vi "CRDS Main.vi"() -> ()   [LabVIEW 2015, in "CRDS.lvclass"]
doc: "This is a basic template for using with children of the instrument class. This provides the basic functionality in a queued state machine. Since the instrument class is abstract, the class must be filled out for meaningful functionality. To get desired behavior, simply swap the instrument class constant in the VIT with a child class that has been properly populated."
uses:
  Main/CRDS.lvclass
  Data/Cell/extparam.ctl
  <vilib>/Utility/error.llb/DialogType.ctl
  Instrument/state.ctl
  Data/Cell/CRDS Cell Data.lvclass/CRDS Cell Data.ctl
  Data/Cell/Read extParam.vi
  <vilib>/Analysis/1siggen.llb/Ramp Pattern by Delta.vi
  Main/Read Data.vi
  Data/Main/Read CellData.vi
  Data/Main/CRDS Data.lvclass
  Data/Cell/CRDS Cell Data.lvclass
  Instrument/Instrument.lvclass
  <vilib>/Analysis/NI_AALBase.lvlib
panel:
  in  "ExpData In":cluster{"A":dbl, "B":dbl, "tau":dbl}[](array[cluster])=[{"A"=16000.0, "B"=100.0, "tau"=60.0}, {"A"=16000.0, "B"=100.0, "tau"=20.0}, {"A"=16000.0, "B"=100.0, "tau"=180.0}]
  out "ExtData":T1[](array[typedef])
  out "taus":cluster{"[0]":dbl, "[1]":dbl, "[2]":dbl}(graph)
  out "tau calc":u32
  in  "Filter":bool
  in  "HK Data":dbl[](array[numeric])
  out "tau_gen":u32
  in  "stop":bool
  out "HK Data":cluster{"[0]":dbl, "[1]":dbl}(graph)
  out "RD Data":dbl[][](graph)
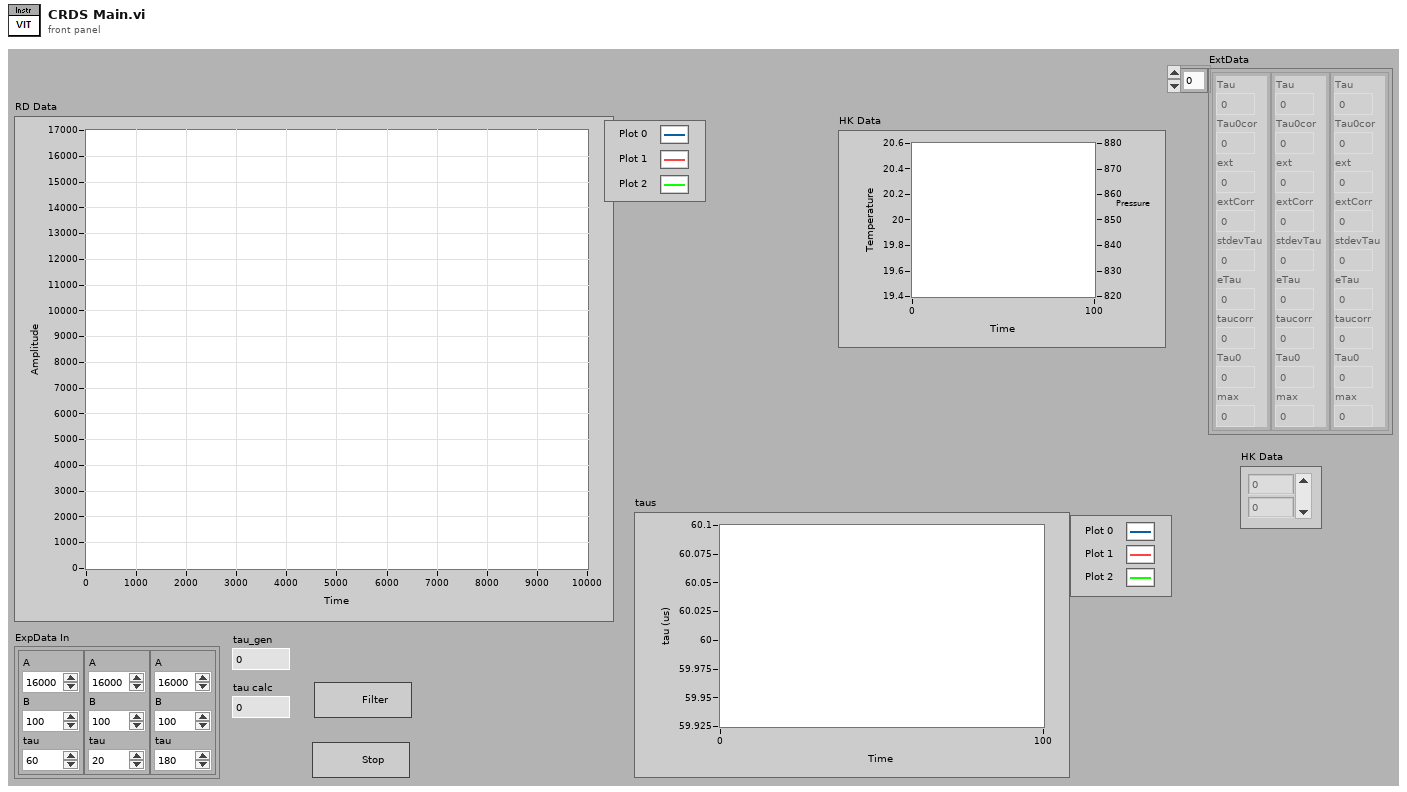
[diagram p1: front panel]
types:
  T1 = typedef "extparam.ctl" = cluster{"Tau":sgl, "Tau0cor":sgl, "ext":sgl, "extCorr":sgl, "stdevTau":sgl, "eTau":sgl, "taucorr":sgl, "Tau0":sgl, "max":sgl}
  T2 = typedef "Instrument.lvclass/state.ctl" = enum8{"Configure", "Acquire", "Wait", "Quit", "Handle Error", "NOOP"}
  T3 = typedef "DialogType.ctl" = u16
  T4 = cluster{"RD Data":dbl[][], "HK Data":dbl[], "Filter":bool}
  T5 = cluster{"RD Data Out":dbl[][], dbl[], "Filter":bool}
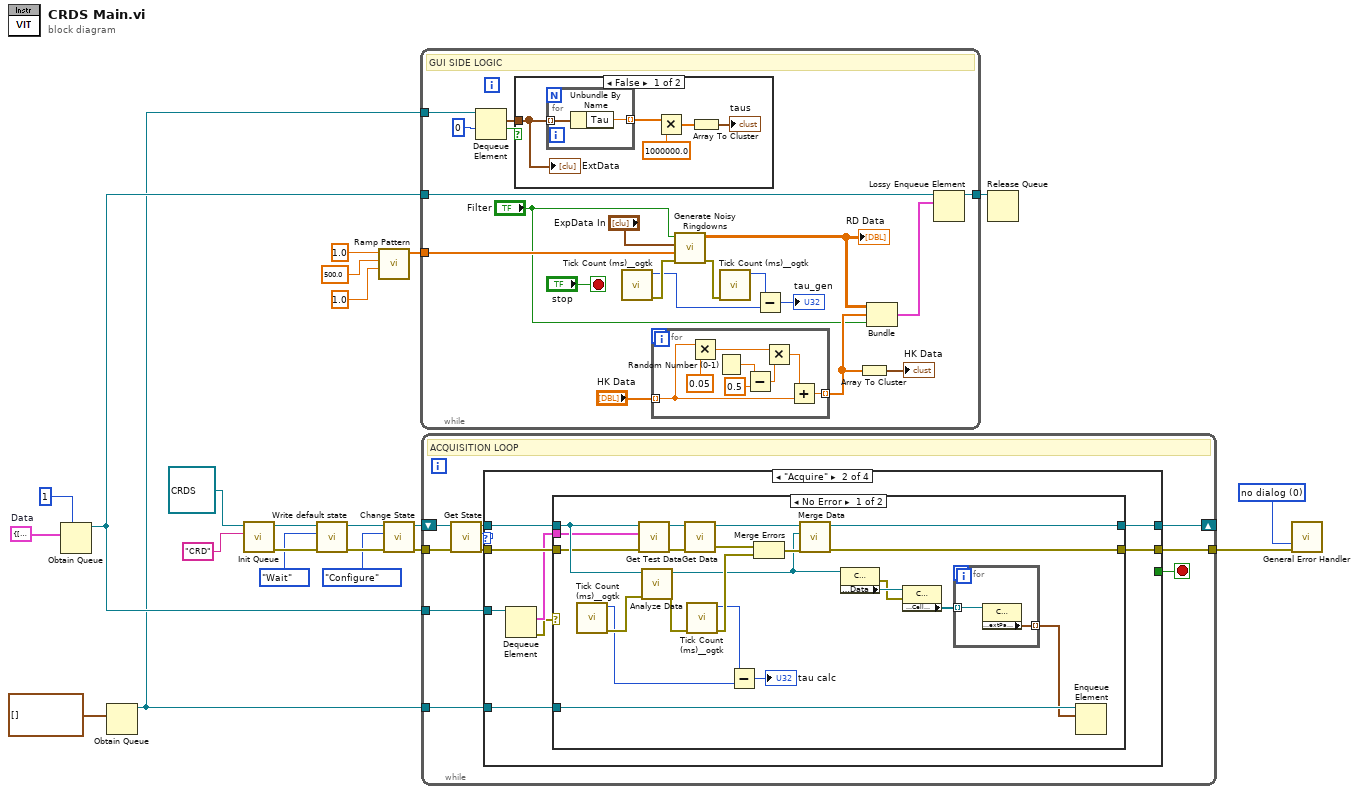
[diagram p0: block diagram]
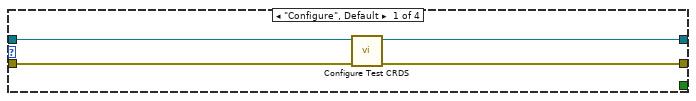
[diagram p2: hidden frame]
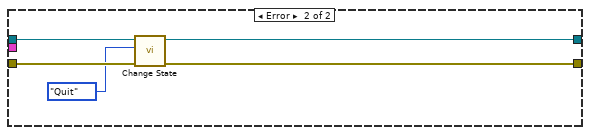
[diagram p3: hidden frame]
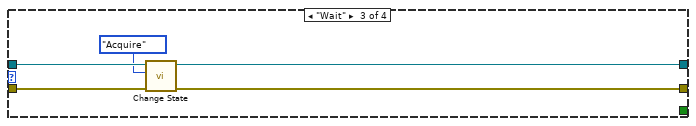
[diagram p4: hidden frame]
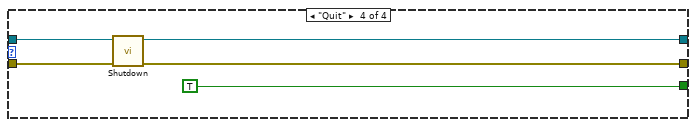
[diagram p5: hidden frame]
diagram:
  w16 = T3 0 items=["no dialog", "OK message", "continue or stop message", "OK message + warnings", "continue/stop + warnings"] ("type of dialog (OK msg:1)")
  w18 = T4 {"RD Data"=[], "HK Data"=[], "Filter"=FALSE}  # Data
  n1 = Obtain Queue(max queue size (-1, unlimited)=1, element data type=w18) -> (queue out=w13:refnum<queue>)  [unwired: 3 in, 2 out]
  n2 = Obtain Queue(element data type=T1[] []) -> (queue out=w1:refnum<queue>)  [unwired: 4 in, 2 out]
  n3 = call "Init Queue.vi"("queue_name"="CRD", "Instrument in"=refnum<class "CRDS.lvclass"> refnum ("CRDS")) -> ("error out"=w10:errorcluster, "Instrument out"=w11:refnum<class "CRDS.lvclass">)  [unwired: 8 in]
  n4 = call "Write default state.vi"("error in (no error)"=w10, "instr state"=state."Wait", "Instrument in"=w11) -> ("error out"=w6:errorcluster, "Instrument out"=w8:refnum<class "CRDS.lvclass">)  [unwired: 7 in]
  n5 = call-poly <vilib>:"Ramp Pattern.vi"("start"=1.0, "end"=500.0, "delta"=1.0) -> ("Ramp Pattern"=w19:dbl[])  [unwired: 6 in, 2 out]
  n6 = call "Change State.vi"("error in"=w6, "instr state"=state."Configure", "Instrument in"=w8) -> ("error out"=w5:errorcluster, "Instrument out"=w7:refnum<class "CRDS.lvclass">)  [unwired: 7 in]
  n7 = while {
    tunnel: w19 -> [w42]
    tunnel: w13 -> [w36]
    tunnel: [w31] -> w12
    tunnel: w1 -> [w28]
    stop <- "stop" stop-if-true
    # "GUI SIDE LOGIC"
    n8 = Dequeue Element(queue=w28, timeout in ms (-1)=0) -> (element=w25:T1[], timed out?=w26:bool)  [unwired: 1 in, 2 out]
    n9 = case shown="False" w26 {
      tunnel: w25 -> [w47 _]
      frame False {
        n10 = for {
          tunnel: w47 -> [w49] mode=indexing
          tunnel: [w48] -> w45 mode=indexing
          n11 = Unbundle By Name(w49) -> ("Tau"=w48:sgl)
        }
        n12 = Multiply(x=w45, y=1000000.0) -> (x*y=w43:dbl[])
        n13 = Array To Cluster(array=w43) -> (cluster=→"taus":cluster{"[0]":dbl, "[1]":dbl, "[2]":dbl})
        "ExtData" <- w47
      }
      frame True {
      }
    }
    n14 = call <userlib>:"Tick Count (ms)__ogtk.vi"() -> ("error out"=w41:errorcluster, "millisecond timer value"=w38:u32)  [unwired: 10 in]
    n15 = for {
      tunnel: "HK Data" -> [w51] mode=indexing
      tunnel: [w50] -> w30 mode=indexing
      n16 = Multiply(x=w51, y=0.05) -> (x*y=w53:dbl)
      n17 = Random Number (0-1)() -> (number: 0 to 1=w56:dbl)
      n18 = Subtract(x=w56, y=0.5) -> (x-y=w54:dbl)
      n19 = Multiply(x=w53, y=w54) -> (x*y=w52:dbl)
      n20 = Add(x=w52, y=w51) -> (x+y=w50:dbl)
    }
    n21 = call "Generate Noisy Ringdowns.vi"("error in"=w41, "Ramp Pattern"=w42, "ExpData In"="ExpData In", "Filter"="Filter") -> ("error out"=w40:errorcluster, "RD Data Out"=w35:dbl[][])  [unwired: 6 in]
    "RD Data" <- w35
    n22 = call <userlib>:"Tick Count (ms)__ogtk.vi"("error in (no error)"=w40) -> ("millisecond timer value"=w39:u32)  [unwired: 9 in, 1 out]
    n23 = Subtract(x=w39, y=w38) -> (x-y=→"tau_gen":u32)
    n24 = Array To Cluster(array=w30) -> (cluster=→"HK Data":cluster{"[0]":dbl, "[1]":dbl})
    n25 = Bundle("RD Data Out"=w35, w30, "Filter"="Filter") -> (w33:T5)  [unwired: 1 in]
    n26 = Lossy Enqueue Element(queue=w36, element=w33) -> (queue out=w31:refnum<queue>)  [unwired: 1 in, 3 out]
  }
  n27 = while "Acquisition" {
    tunnel: w5 -> [w67]
    shift-right: [w61] -> _
    shift-left: w7 -> [w65]
    tunnel: [w60] -> w17
    tunnel: w13 -> [w59]
    tunnel: w1 -> [w58]
    stop <- w62 stop-if-true
    # "ACQUISITION LOOP"
    n28 = call "Get State.vi"("error in"=w67, "Instrument in"=w65) -> ("error out"=w63:errorcluster, "default state"=w66:T2, "Instrument out"=w64:refnum<class "CRDS.lvclass">)  [unwired: 7 in]
    n29 = case shown="\"Acquire\"" w66 {
      tunnel: w64 -> [w71 w76 w113 w117]
      tunnel: w63 -> [w70 w79 w112 w116]
      tunnel: [_ _ _ TRUE] -> w62
      tunnel: [w69 w78 w111 w115] -> w61
      tunnel: [w68 w77 w110 w114] -> w60
      tunnel: w59 -> [_ w75 _ _]
      tunnel: w58 -> [_ w72 _ _]
      frame "Configure", Default {
        n30 = call "Configure Test CRDS.vi"("error in (no error)"=w70, "CRDS in"=w71) -> ("error out"=w68:errorcluster, "CRDS out"=w69:refnum<class "CRDS.lvclass">)  [unwired: 8 in]
      }
      frame "Acquire" {
        n31 = Dequeue Element(queue=w75) -> (element=w74:T4, error out=w73:errorcluster)  [unwired: 2 in, 2 out]
        n32 = case shown="No Error" w73 {
          tunnel: w79 -> [w82 w107]
          tunnel: [w99 w106] -> w78
          tunnel: [w97 w105] -> w77
          tunnel: w76 -> [w96 w108]
          tunnel: w74 -> [w94 _]
          tunnel: w72 -> [w84 _]
          frame No Error {
            n33 = call <userlib>:"Tick Count (ms)__ogtk.vi"() -> ("error out"=w91:errorcluster, "millisecond timer value"=w89:u32)  [unwired: 10 in]
            n34 = call "Get Test Data.vi"("error in"=w82, "Data"=w94, "CRDS in"=w96) -> ("error out"=w81:errorcluster, "CRDS out"=w95:refnum<class "CRDS.lvclass">)  [unwired: 7 in]
            n35 = call-dynamic "Analyze Data.vi"("error in"=w91, "CRDS in"=w96) -> ("error out"=w93:errorcluster, "CRDS out"=w87:refnum<class "CRDS.lvclass">)  [unwired: 8 in]
            n36 = call-dynamic "Get Data.vi"("error in"=w81, "CRDS in"=w95) -> ("error out"=w101:errorcluster, "CRDS out"=w100:refnum<class "CRDS.lvclass">)  [unwired: 8 in]
            n37 = call <userlib>:"Tick Count (ms)__ogtk.vi"("error in (no error)"=w93) -> ("error out"=w92:errorcluster, "millisecond timer value"=w90:u32)  [unwired: 9 in]
            n38 = Subtract(x=w90, y=w89) -> (x-y=→"tau calc":u32)
            n39 = Merge Errors(w101, w92) -> (w98:errorcluster)
            n40 = call-dynamic "Merge Data.vi"("error in"=w98, "Analyzed"=w87, "Acquired"=w100) -> ("error out"=w97:errorcluster, "CRDS out"=w99:refnum<class "CRDS.lvclass">)  [unwired: 7 in]
            n41 = property class="CRDS"(reference=w87) -> (error out=w80:errorcluster, "Data Access:Data"=w86:refnum<class "CRDS Data.lvclass">)  [unwired: 1 in, 1 out]
            n42 = property class="CRDS"(reference=w86, error in=w80) -> ("Data Access:Cell Data"=w85:refnum<class "CRDS Cell Data.lvclass">[])  [unwired: 2 out]
            n43 = for {
              tunnel: w85 -> [w103] mode=indexing
              tunnel: [w102] -> w83 mode=indexing
              n44 = property class="CRDS Cell"(reference=w103) -> ("Data Access:extParam"=w102:T1)  [unwired: 1 in, 2 out]
            }
            n45 = Enqueue Element(queue=w84, element=w83) -> ()  [unwired: 2 in, 3 out]
          }
          frame Error {
            n46 = call "Change State.vi"("error in"=w107, "instr state"=state."Quit", "Instrument in"=w108) -> ("error out"=w105:errorcluster, "Instrument out"=w106:refnum<class "CRDS.lvclass">)  [unwired: 7 in]
          }
        }
      }
      frame "Wait" {
        n47 = call "Change State.vi"("error in"=w112, "instr state"=state."Acquire", "Instrument in"=w113) -> ("error out"=w110:errorcluster, "Instrument out"=w111:refnum<class "CRDS.lvclass">)  [unwired: 7 in]
      }
      frame "Quit" {
        n48 = call-dynamic "Shutdown.vi"("error in"=w116, "Instrument in"=w117) -> ("error out"=w114:errorcluster, "Instrument out"=w115:refnum<class "CRDS.lvclass">)  [unwired: 8 in]
      }
    }
  }
  n49 = Release Queue(queue=w12) -> ()  [unwired: 2 in, 3 out]
  n50 = call <vilib>:"General Error Handler.vi"("type of dialog (OK msg:1)"=w16, "error in (no error)"=w17) -> ()  [unwired: 9 in, 5 out]
